vi "Launch VI.vi"(8 "error in (no error)":errorcluster, 10 "Stop Button":bool, 11 "vi path":path=path "C:/Program Files (x86)/National Instruments/LabVIEW 2014/vi.lib/Utility/visa.llb/Open VISA Session Monitor.vi") -> (0 "error out":errorcluster)   [LabVIEW 2014]
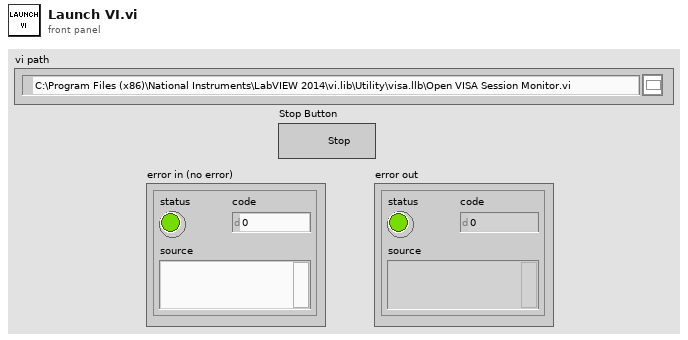
[diagram p1: front panel]
types:
  T1 = enum32{"Invalid", "Standard", "Closed", "Hidden", "Minimized", "Maximized"}
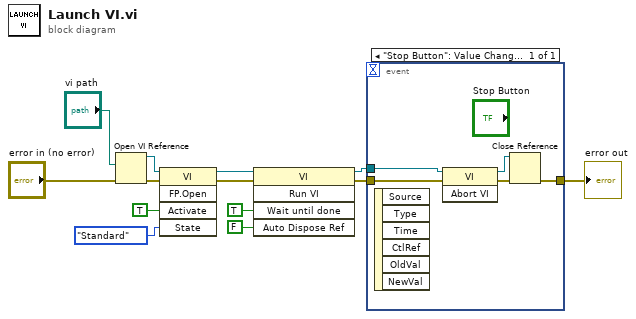
[diagram p0: block diagram]
diagram:
  n1 = Open VI Reference(vi path="vi path", error in (no error)="error in (no error)") -> (vi reference=w13:refnum<vi>, error out=w8:errorcluster)  [unwired: 4 in]
  n2 = invoke class="VI" method="FP.Open"(reference=w13, error in=w8, "Activate"=TRUE ("Activate?"), "State"=T1."Standard") -> (reference out=w10:refnum<vi>, error out=w9:errorcluster)  [unwired: 1 in, 3 out]
  n3 = invoke class="VI" method="Run VI"(reference=w10, error in=w9, "Wait until done"=TRUE ("Wait Until Done"), "Auto Dispose Ref"=FALSE ("Auto Dispose Reference")) -> (reference out=w5:refnum<vi>, error out=w4:errorcluster)  [unwired: 1 in, 3 out]
  n4 = event shown="[0] \"Stop Button\": Value Change" {
    selector: _ -> [_]
    dyn-events: _ -> [_]
    timeout: _ -> [_]
    tunnel: w5 -> [w17]
    tunnel: w4 -> [w16]
    tunnel: [w18] -> w3
    event "Stop Button": Value Change {
      n5 = event-data() -> ()  [unwired: 1 in, 6 out]
      n6 = invoke class="VI" method="Abort VI"(reference=w17, error in=w16) -> (reference out=w15:refnum<vi>, error out=w14:errorcluster)  [unwired: 1 in, 1 out]
      n7 = Close Reference(reference=w15, error in (no error)=w14) -> (error out=w18:errorcluster)
    }
  }
  "error out" <- w3
